vi "Config Reference Point.vi"(6 "Loss Single (off)":bool, 7 "Capacitance Single (off)":bool, 8 "error in":errorcluster, 9 "Loss Point (0 jpF)":dbl min=-99999999.0 max=99999999.0 format="%#_10f", 10 "Capacitance Point (0 pF)":dbl min=-99999999.0 max=99999999.0 format="%#_10f", 11 "VISA resource name":refnum<visa-resource-name>) -> (0 "error out":errorcluster, 3 "VISA resource name out":refnum<visa-resource-name>)   [LabVIEW 2016, in "Andeen-Hagerling 2550.lvlib"]
doc: "This VI provides manual and automatic ways to enter capacitance and/or loss Reference values. When Capacitance/Loss single switches are set to ON, the last measured values are used as the reference values. When the single switches are set to off, the manually entered Reference Point values are used."
uses:
  Andeen-Hagerling 2550.lvlib
panel:
  # "Reference Point"
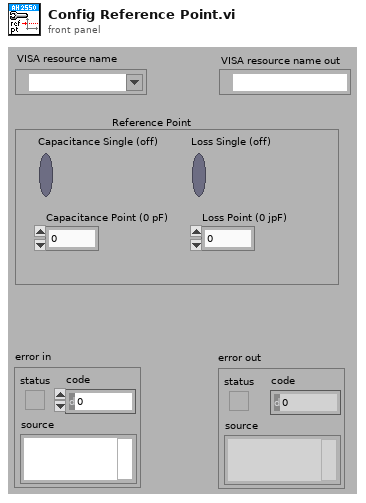
[diagram p1: front panel]
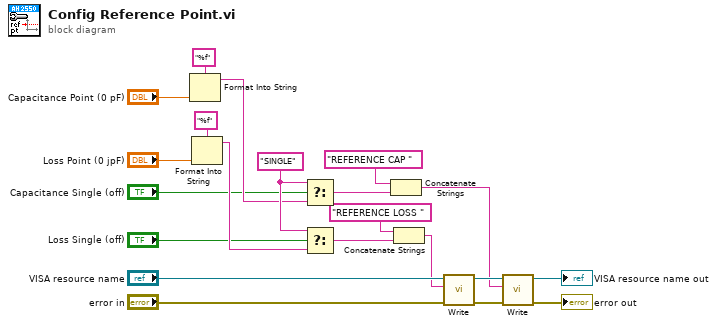
[diagram p0: block diagram]
diagram:
  w15 = "SINGLE" ("format string")
  n1 = Format Into String(format string="%f", "Capacitance Point (0 pF)") -> (resulting string=w14:string)  [unwired: 2 in, 1 out]
  n2 = Format Into String(format string="%f", "Loss Point (0 jpF)") -> (resulting string=w13:string)  [unwired: 2 in, 1 out]
  n3 = Select(t=w15, s="Capacitance Single (off)", f=w14) -> (s? t:f=w9:string)
  n4 = Select(t=w15, s="Loss Single (off)", f=w13) -> (s? t:f=w8:string)
  n5 = Concatenate Strings("REFERENCE CAP " ("format string"), w9) -> (w1:string)
  n6 = Concatenate Strings("REFERENCE LOSS " ("format string"), w8) -> (w2:string)
  n7 = call "Write.vi"("error in"="error in", "command"=w2, "VISA resource name"="VISA resource name") -> ("error out"=w3:errorcluster, "VISA resource name out"=w5:refnum<visa-resource-name>)  [unwired: 7 in]
  n8 = call "Write.vi"("error in"=w3, "command"=w1, "VISA resource name"=w5) -> ("error out"=→"error out":errorcluster, "VISA resource name out"=→"VISA resource name out":refnum<visa-resource-name>)  [unwired: 7 in]
